vi "Get All Controls Tip Strips.vi"(8 "Error In":errorcluster, 11 "VI Ref":refnum<vi>) -> (0 "Error Out":errorcluster, 3 "Controls Tip Strips":string[](array[string]))   [LabVIEW 2021]
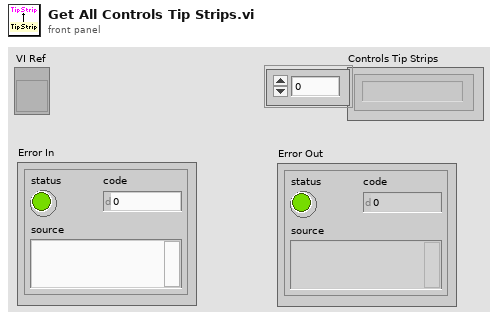
[diagram p1: front panel]
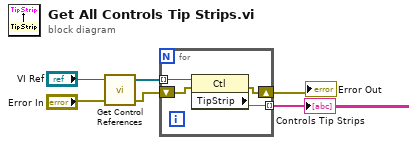
[diagram p0: block diagram]
diagram:
  n1 = call "Get Control References.vi"("error in"="Error In", "VI  Ref"="VI Ref") -> ("error out"=w2:errorcluster, "Controls[]"=w4:refnum<vi>[])  [unwired: 1 in, 1 out]
  n2 = for {
    tunnel: w4 -> [w10] mode=indexing
    tunnel: [w9] -> w6 mode=indexing
    shift-right: [w7] -> w1
    shift-left: w2 -> [w8]
    n3 = property class="Ctl"(reference=w10, error in=w8) -> (error out=w7:errorcluster, "TipStrip"=w9:string)  [unwired: 1 out]
  }
  "Controls Tip Strips" <- w6
  "Error Out" <- w1
